vi "Actor Core.vi"(8 "error in":errorcluster, 11 "Unit_Test_NI6008 in":refnum<class "Unit_Test_NI6008.lvclass">) -> (0 "error out":errorcluster, 3 "Actor out":refnum<class "Actor.lvclass">)   [LabVIEW 2020, in "Unit_Test_NI6008.lvlib" / "Unit_Test_NI6008.lvclass"]
doc: "(<B>Filename</B>: Actor Framework.lvlib:Actor.lvclass:Actor Core.vi)\n\nReceives messages to the actor, reacts to them, and initiates any error handling that may shut the actor down.\n\nDescendant classes may override this VI to append parallel tasks for the actor to complete while it handles messages. Overrides use the Call Parent Class Method node."
uses:
  Unit_Test_NI6008.lvclass
  C:/Program Files/National Instruments/LabVIEW 2020/vi.lib/ActorFramework/Actor/Actor.lvclass
  <vilib>/ActorFramework/Actor/Actor.lvclass
  Actor_NI6008/Actor_NI6008/Actor_NI6008.lvclass
  Unit_Test_NI6008.lvclass/Unit_Test_NI6008.ctl
  <vilib>/ActorFramework/Actor/Actor.lvclass/Actor.ctl
  <vilib>/ActorFramework/Message Enqueuer/Message Enqueuer.lvclass/Message Enqueuer.ctl
  <vilib>/ActorFramework/Stop Msg/Stop Msg.lvclass/Stop Msg.ctl
  Actor_NI6008/Actor_NI6008 Messages/NI6008 DUT Switch Msg/NI6008 DUT Switch Msg.lvclass/NI6008 DUT Switch Msg.ctl
  3eb12a7e-eef2-44c0-8e94-63c820516bea.vi
  <vilib>/ActorFramework/Message Enqueuer/Init from Existing Queue.vi
  <vilib>/ActorFramework/Stop Msg/Send Emergency Stop.vi
  <vilib>/ActorFramework/Stop Msg/Send Normal Stop.vi
  <vilib>/ActorFramework/Message Enqueuer/Enqueue.vi
  <vilib>/ActorFramework/Message Enqueuer/Enqueue Critical.vi
  <vilib>/ActorFramework/Stop Msg/Stop Msg.lvclass
  C:/Program Files/National Instruments/LabVIEW 2020/vi.lib/ActorFramework/Message/Message.lvclass
  Actor_NI6008/Actor_NI6008 Messages/NI6008 DUT Switch Msg/NI6008 DUT Switch Msg.lvclass
  <vilib>/ActorFramework/Message Priority Queue/Priority Enqueue.vi
  <vilib>/ActorFramework/Message Enqueuer/Message Enqueuer.lvclass
  <vilib>/Comparison/Equal/Equal Functor/Equal Functor.lvclass
panel:
  out "log":string[](array[string])
  in  "DUT Channel":T1
  # "NI6008 Unit Test Front Panel"
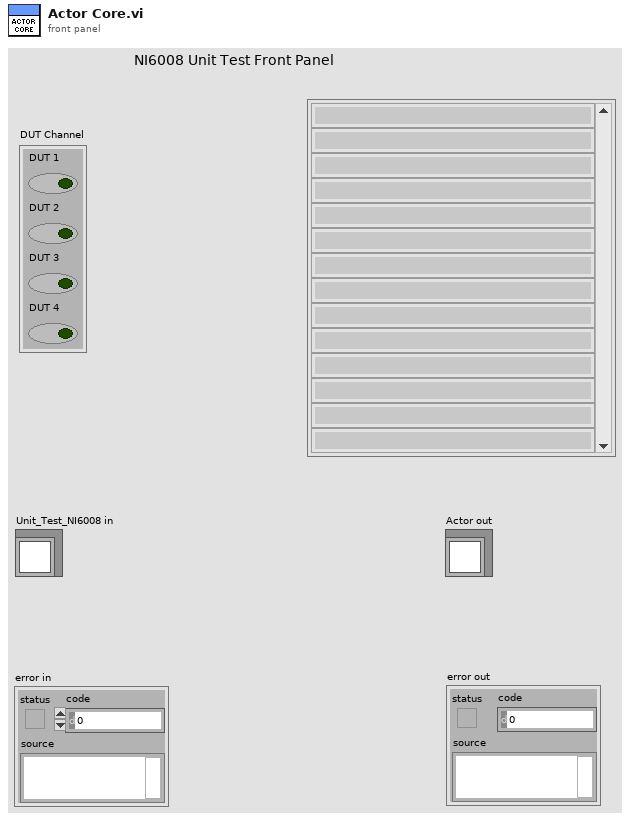
[diagram p1: front panel]
types:
  T1 = cluster{"DUT 1":bool, "DUT 2":bool, "DUT 3":bool, "DUT 4":bool}
  T2 = enum32{"Invalid", "Standard", "Closed", "Hidden", "Minimized", "Maximized"}
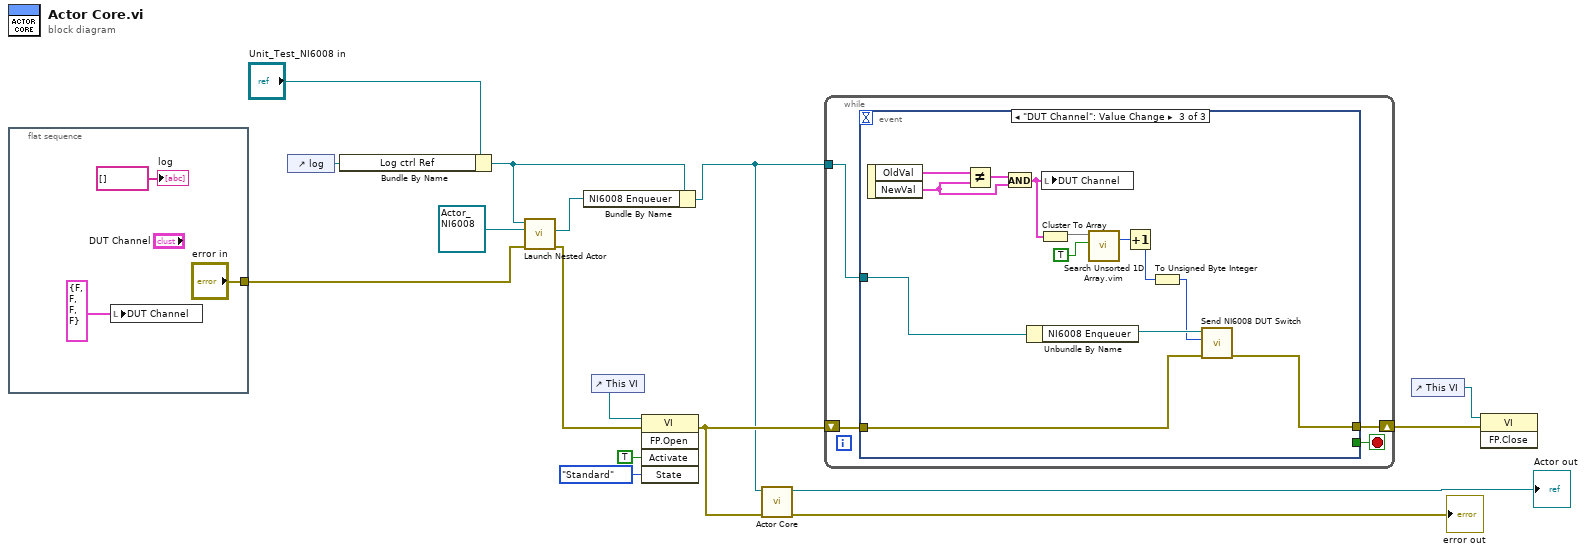
[diagram p0: block diagram]
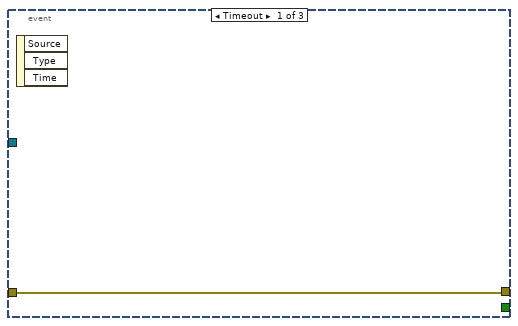
[diagram p2: hidden frame]
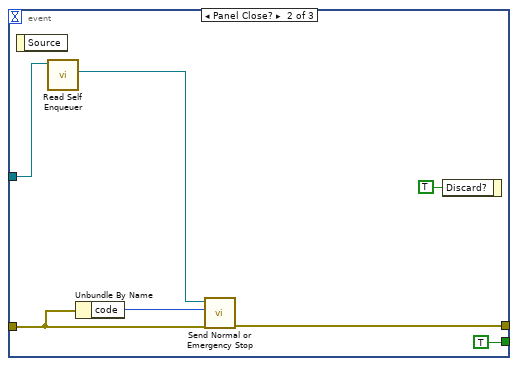
[diagram p3: hidden frame]
diagram:
  n1 = flat-sequence {
    tunnel: ["error in"] -> w1
    frame #0 {
      n2 = local write "DUT Channel"(T1 {"DUT 1"=FALSE, "DUT 2"=FALSE, "DUT 3"=FALSE, "DUT 4"=FALSE} ("DUT Channel")) -> ()
      "log" <- string[] [] ("log")
    }
  }
  n3 = control-ref of="log"() -> (w3:refnum<vi>)
  n4 = Bundle By Name(cluster="Unit_Test_NI6008 in", "Log ctrl Ref"=w3) -> (w2:refnum<class "Unit_Test_NI6008.lvclass">)
  n5 = call <vilib>:"Launch Nested Actor.vi"("error in (no error)"=w1, "Nested Actor"=refnum<class "Actor_NI6008.lvclass"> refnum ("Actor_NI6008.lvlib:Actor_NI6008.lvclass"), "Caller Actor in"=w2) -> ("error out"=w5:errorcluster, "Nested Actor's Enqueuer"=w7:refnum<class "Message Enqueuer.lvclass">)  [unwired: 6 in, 1 out]
  n6 = Bundle By Name(cluster=w2, "NI6008 Enqueuer"=w7) -> (w6:refnum<class "Unit_Test_NI6008.lvclass">)
  n7 = control-ref of="This VI"() -> (w12:refnum<vi>)
  n8 = invoke class="VI" method="FP.Open"(reference=w12, error in=w5, "Activate"=TRUE ("Activate?"), "State"=T2."Standard") -> (error out=w9:errorcluster)  [unwired: 1 in, 4 out]
  n9 = call-parent "Actor Core.vi"("error in"=w9, "Actor in"=w6) -> ("error out"=→"error out":errorcluster, "Actor out"=→"Actor out":refnum<class "Actor.lvclass">)  [unwired: 8 in]
  n10 = while {
    tunnel: w6 -> [w22]
    shift-right: [w20] -> w14
    shift-left: w9 -> [w21]
    stop <- w23 stop-if-true
    n11 = event shown="[2] \"DUT Channel\": Value Change" {
      selector: _ -> [_ _ _]
      dyn-events: _ -> [_ _ _]
      timeout: _ -> [_ _ _]
      tunnel: [_ TRUE ("Discard?") _] -> w23
      tunnel: w22 -> [_ w29 w41]
      tunnel: w21 -> [w24 w28 w33]
      tunnel: [w24 w25 w32] -> w20
      event Timeout {
        n12 = event-data() -> ()  [unwired: 1 in, 3 out]
      }
      event Panel Close? {
        n13 = event-data() -> ()  [unwired: 1 in, 1 out]
        n14 = call <vilib>:"Read Self Enqueuer.vi"("Actor"=w29) -> ("Self Enqueuer"=w26:refnum<class "Message Enqueuer.lvclass">)  [unwired: 10 in]
        n15 = Unbundle By Name(w28) -> ("code"=w27:i32)
        n16 = call <vilib>:"Send Normal or Emergency Stop.vi"("error in (no error)"=w28, "final error code"=w27, "Message Enqueuer"=w26) -> ("error out"=w25:errorcluster)  [unwired: 8 in]
        n17 = event-data("Discard?"=TRUE) -> ()  [unwired: 1 in, 1 out]
      }
      event "DUT Channel": Value Change {
        n18 = event-data() -> ("OldVal"=w44:T1, "NewVal"=w42:T1)  [unwired: 1 in]
        n19 = Not Equal?(x=w44, y=w42) -> (x != y?=w43:T1)
        n20 = And(x=w43, y=w42) -> (x .and. y?=w39:T1)
        n21 = Unbundle By Name(w41) -> ("NI6008 Enqueuer"=w40:refnum<class "Message Enqueuer.lvclass">)
        n22 = Cluster To Array(cluster=w39) -> (array=w36:bool[])
        n23 = local write "DUT Channel"(w39) -> ()
        n24 = call "Search Unsorted 1D Array.vim"("element"=TRUE, "unsorted 1D array"=w36) -> ("index of element"=w38:i32)  [unwired: 9 in]
        n25 = Increment(x=w38) -> (x+1=w35:i32)
        n26 = To Unsigned Byte Integer(number=w35) -> (unsigned 8bit integer=w34:u8)
        n27 = call "Send NI6008 DUT Switch.vi"("error in (no error)"=w33, "DUT No."=w34, "Message Enqueuer"=w40) -> ("error out"=w32:errorcluster)  [unwired: 7 in, 1 out]
      }
    }
  }
  n28 = control-ref of="This VI"() -> (w13:refnum<vi>)
  n29 = invoke class="VI" method="FP.Close"(reference=w13, error in=w14) -> ()  [unwired: 1 in, 3 out]
